vi "Example.vi"(8 "error in (no error)":errorcluster, 11 "Input":string="\u0011S\u0007\r\r\u0011W\u0007") -> (0 "error out":errorcluster, 3 "Key Array":T1(array[cluster]))   [LabVIEW 2015]
panel:
  in  "String":string
  out "Key 2":u8(ring)=65
  in  "Key":u8(ring)=65
  out "unsigned byte array":u8[](array[numeric])
  # "This VI is an example that uses simulated Key Presses to \ntype into a String control programmatically.  They Key Array \ncontrol is what defines which keys are pressed and for how\nlong.  Note that the shift key is pushed down and up in \nseparate steps and that the alphabetical keys are pressed.\nThis is equivalent to holding the shift key down while pressing\n'H', the result being an uppercase 'H'.\n\nSimply run this VI and 'Hello' will be programmatically typed in\nthe above Output box."
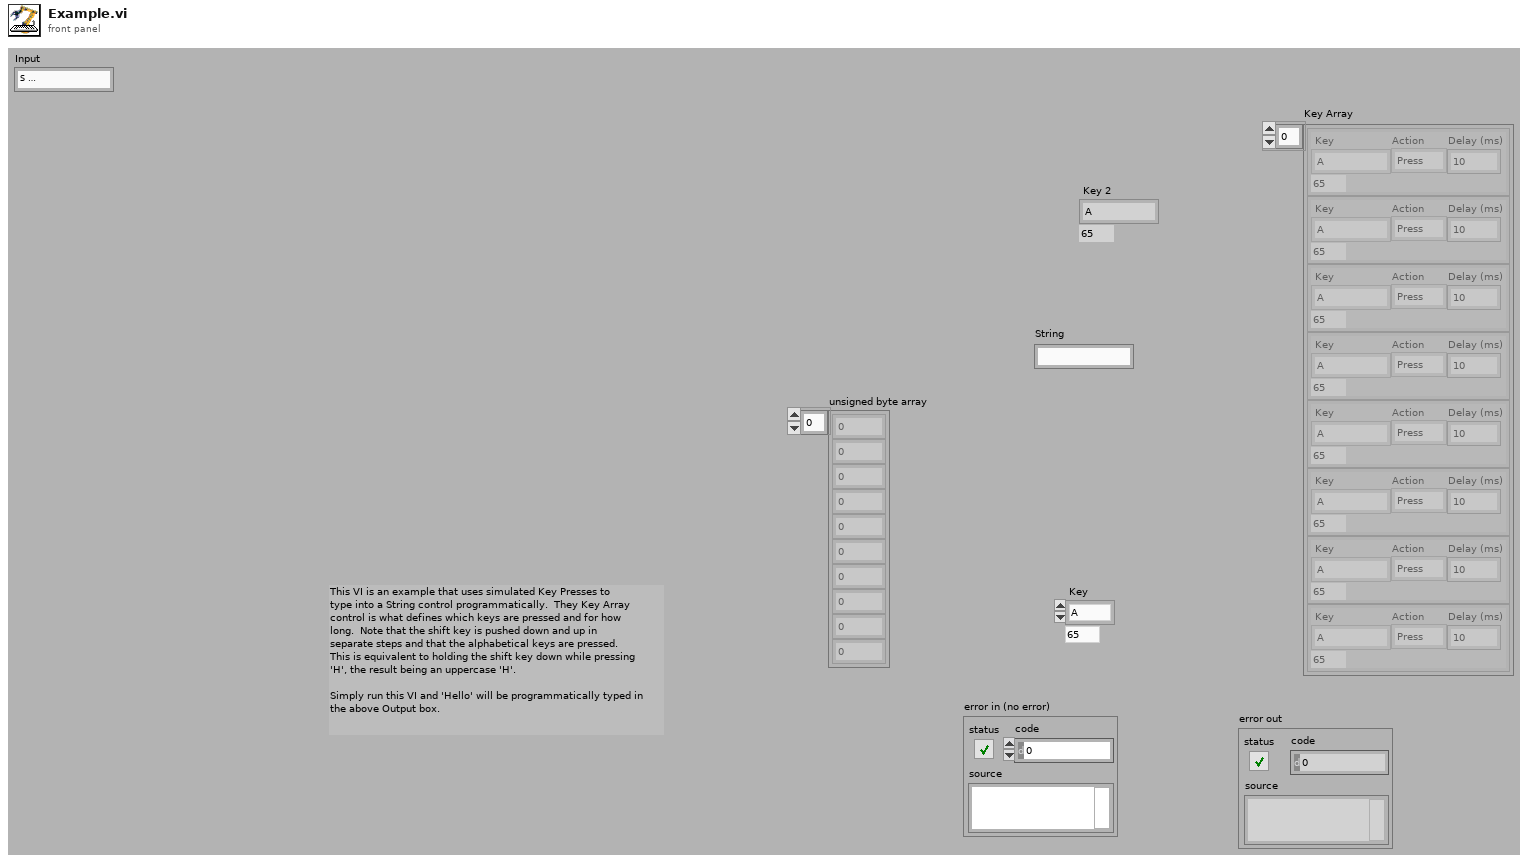
[diagram p1: front panel]
types:
  T1 = cluster{" Key":u8, "Action":enum16{"Press", "Up", "Down"}, "Delay (ms)":u32}[]
  T2 = cluster{" Key":u8, "Action":enum16{"Press", "Up", "Down"}, "Delay (ms)":u32}
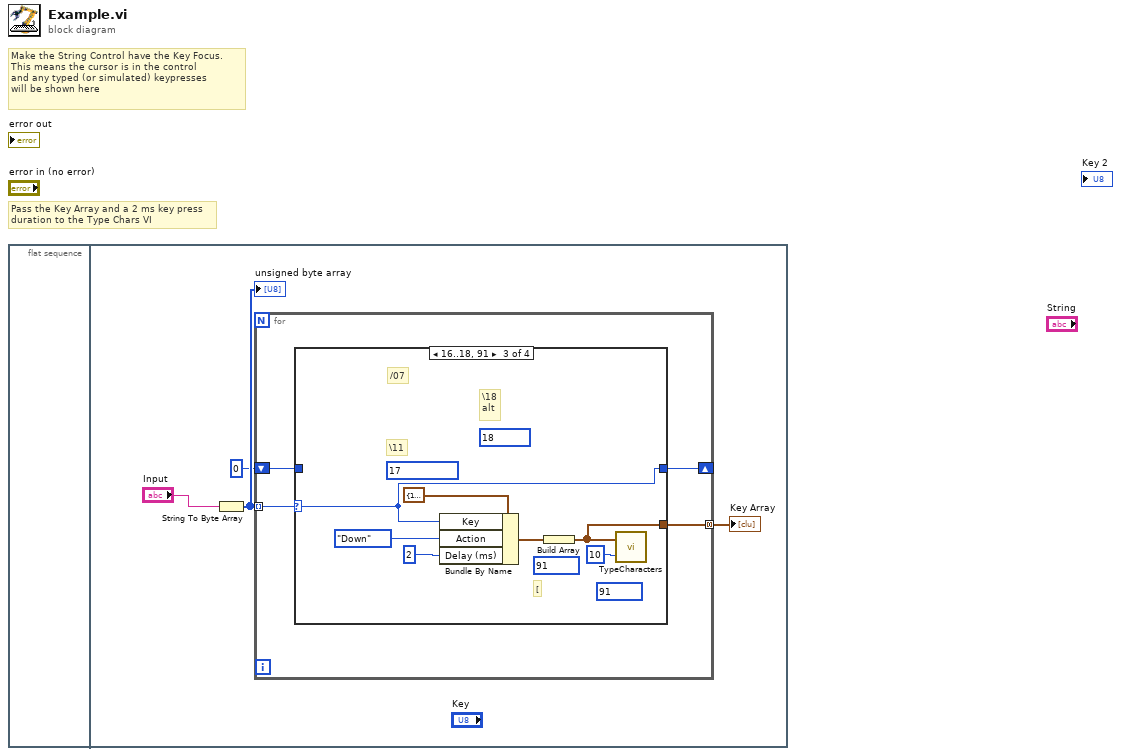
[diagram p0: block diagram]
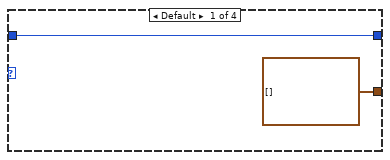
[diagram p2: hidden frame]
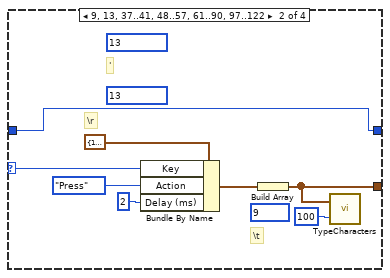
[diagram p3: hidden frame]
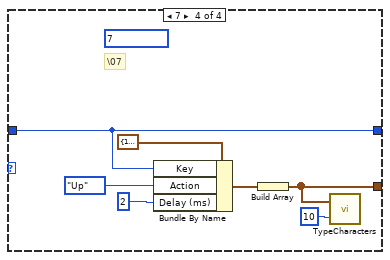
[diagram p4: hidden frame]
diagram:
  # "Pass the Key Array and a 2 ms key press\nduration to the Type Chars VI"
  # "Make the String Control have the Key Focus.\nThis means the cursor is in the control\nand any typed (or simulated) keypresses\nwill be shown here"
  n1 = flat-sequence {
    frame #0 {
    }
    frame #1 {
      n2 = String To Byte Array(string="Input") -> (unsigned byte array=w4:u8[])
      "unsigned byte array" <- w4
      n3 = for {
        tunnel: w4 -> [w8] mode=indexing
        shift-right: [w7] -> _
        shift-left: u8 0 -> [w6]
        tunnel: [w5] -> w1 mode=concatenating
        n4 = case shown="16..18, 91" w8 {
          selector: w8 -> [_ w17 w20 _]
          tunnel: [w10 w12 w20 w27] -> w7
          tunnel: w6 -> [w10 w12 _ w27]
          tunnel: [T1 [] w11 w19 w26] -> w5
          frame Default {
          }
          frame 9, 13, 37..41, 48..57, 61..90, 97..122 {
            (unwired) u8 13 ("Key")
            (unwired) u8 13 ("Key")
            (unwired) u8 9 ("Key")
            # "\\r"
            # "'"
            # "\\t"
            n5 = Bundle By Name(cluster=T2 {" Key"=17, "Action"=enum."Down", "Delay (ms)"=10} ("Cluster"), "Key"=w17, "Action"=enum16{"Press", "Up", "Down"}."Press", "Delay (ms)"=u32 2) -> (w13:T2)
            n6 = Build Array(w13) -> (w11:T1)
            n7 = call "TypeCharacters.vi"("Length of Key Press (ms)"=u32 100, "Key Array"=w11) -> ()  [unwired: 1 in]
          }
          frame 16..18, 91 {
            (unwired) u8 18 ("Key")
            (unwired) u8 91 ("Key")
            (unwired) u8 91 ("Key")
            (unwired) u8 17 ("Key")
            # "\\18\nalt"
            # "["
            # "\\11"
            # "/07"
            n8 = Bundle By Name(cluster=T2 {" Key"=17, "Action"=enum."Down", "Delay (ms)"=10} ("Cluster"), "Key"=w20, "Action"=enum16{"Press", "Up", "Down"}."Down", "Delay (ms)"=u32 2) -> (w24:T2)
            n9 = Build Array(w24) -> (w19:T1)
            n10 = call "TypeCharacters.vi"("Length of Key Press (ms)"=u32 10, "Key Array"=w19) -> ()  [unwired: 1 in]
          }
          frame 7 {
            (unwired) u8 7 ("Key")
            # "\\07"
            n11 = Bundle By Name(cluster=T2 {" Key"=17, "Action"=enum."Down", "Delay (ms)"=10} ("Cluster"), "Key"=w27, "Action"=enum16{"Press", "Up", "Down"}."Up", "Delay (ms)"=u32 2) -> (w31:T2)
            n12 = Build Array(w31) -> (w26:T1)
            n13 = call "TypeCharacters.vi"("Length of Key Press (ms)"=u32 10, "Key Array"=w26) -> ()  [unwired: 1 in]
          }
        }
      }
      "Key Array" <- w1
    }
  }
